vi "labpavi4.vi"() -> ()   [LabVIEW 2025]
uses:
  <vilib>/Analysis/3filter.llb/Filter Passband Type.ctl
  <vilib>/Analysis/2dsp.llb/Real FFT.vi
  <vilib>/Analysis/3filter.llb/Butterworth Filter (DBL).vi
  <vilib>/measure/NI_MABase.lvlib
  <vilib>/Analysis/NI_AALPro.lvlib
  <vilib>/Analysis/NI_AALBase.lvlib
panel:
  out "Waveform Graph 3":dbl[](graph)
  out "Waveform Graph":dbl[](graph)
  in  "samples":dbl=10.0 format="%0.2p"
  in  "sampfreq":dbl=10.0 format="%0.2p"
  out "Frequency label":waveform(dbl)(graph)
  out "spectrum":cluster{"Y":dbl[], "Y":dbl[]}[](graph)
  in  "deltaf":dbl
  out "Output":dbl[](graph)
  in  "fc":dbl
  out "Message":waveform(dbl)(graph)
  in  "fm":dbl=10.0 format="%0.2p"
  in  "am":dbl=1.0 format="%0.2p"
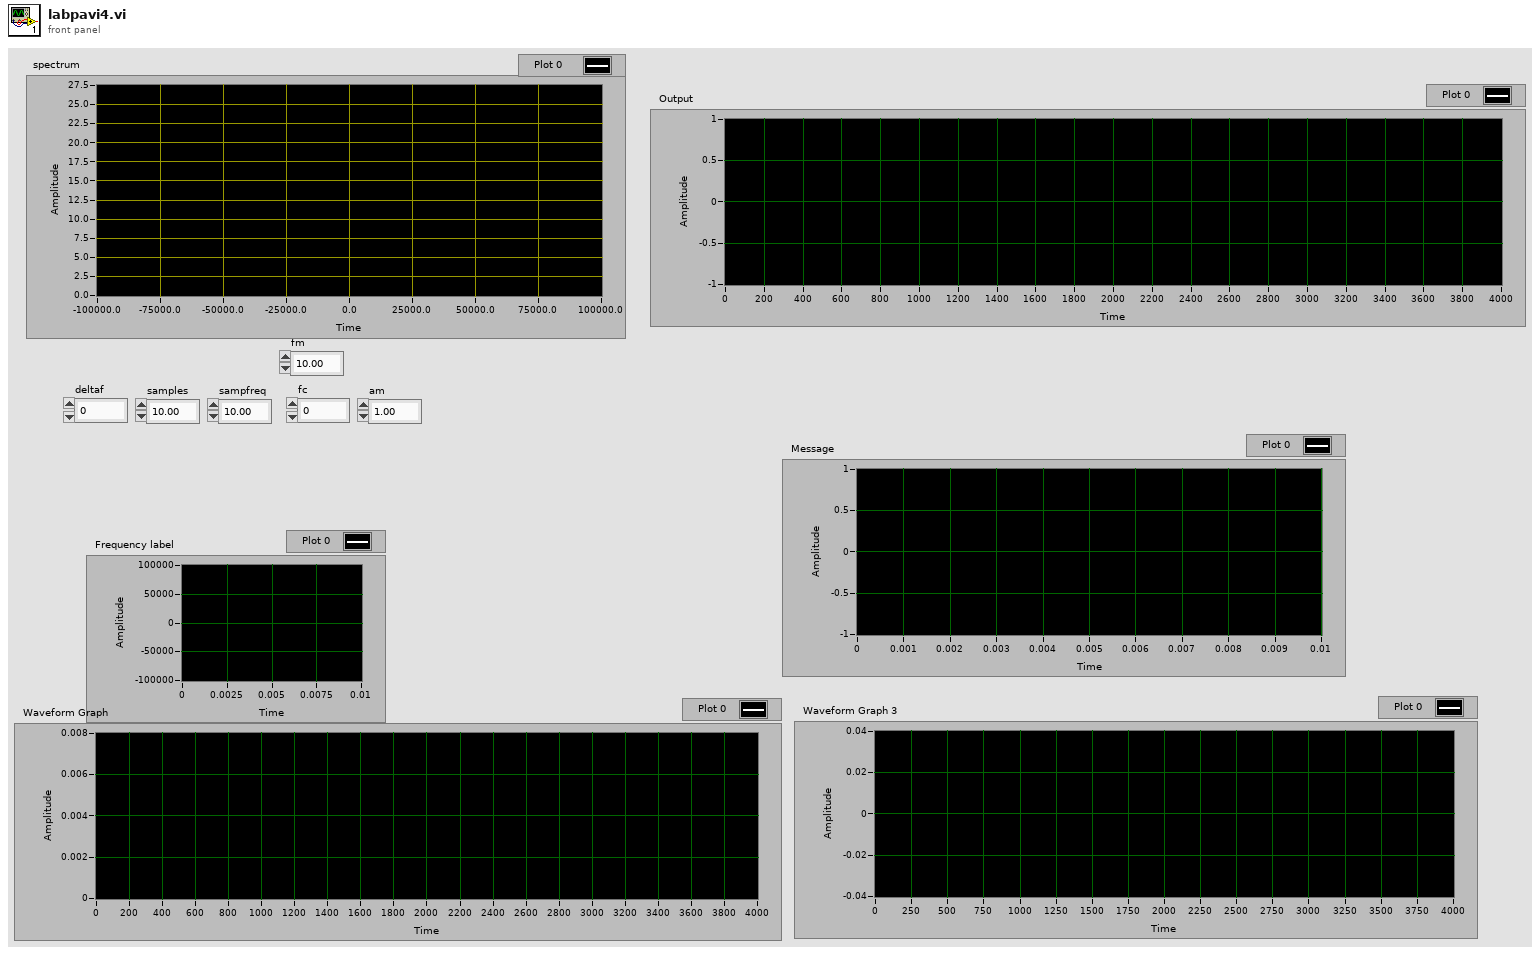
[diagram p1: front panel]
types:
  T1 = typedef "NI_AALBase.lvlib/Filter Passband Type.ctl" = enum32{"Lowpass", "Highpass", "Bandpass", "Bandstop"}
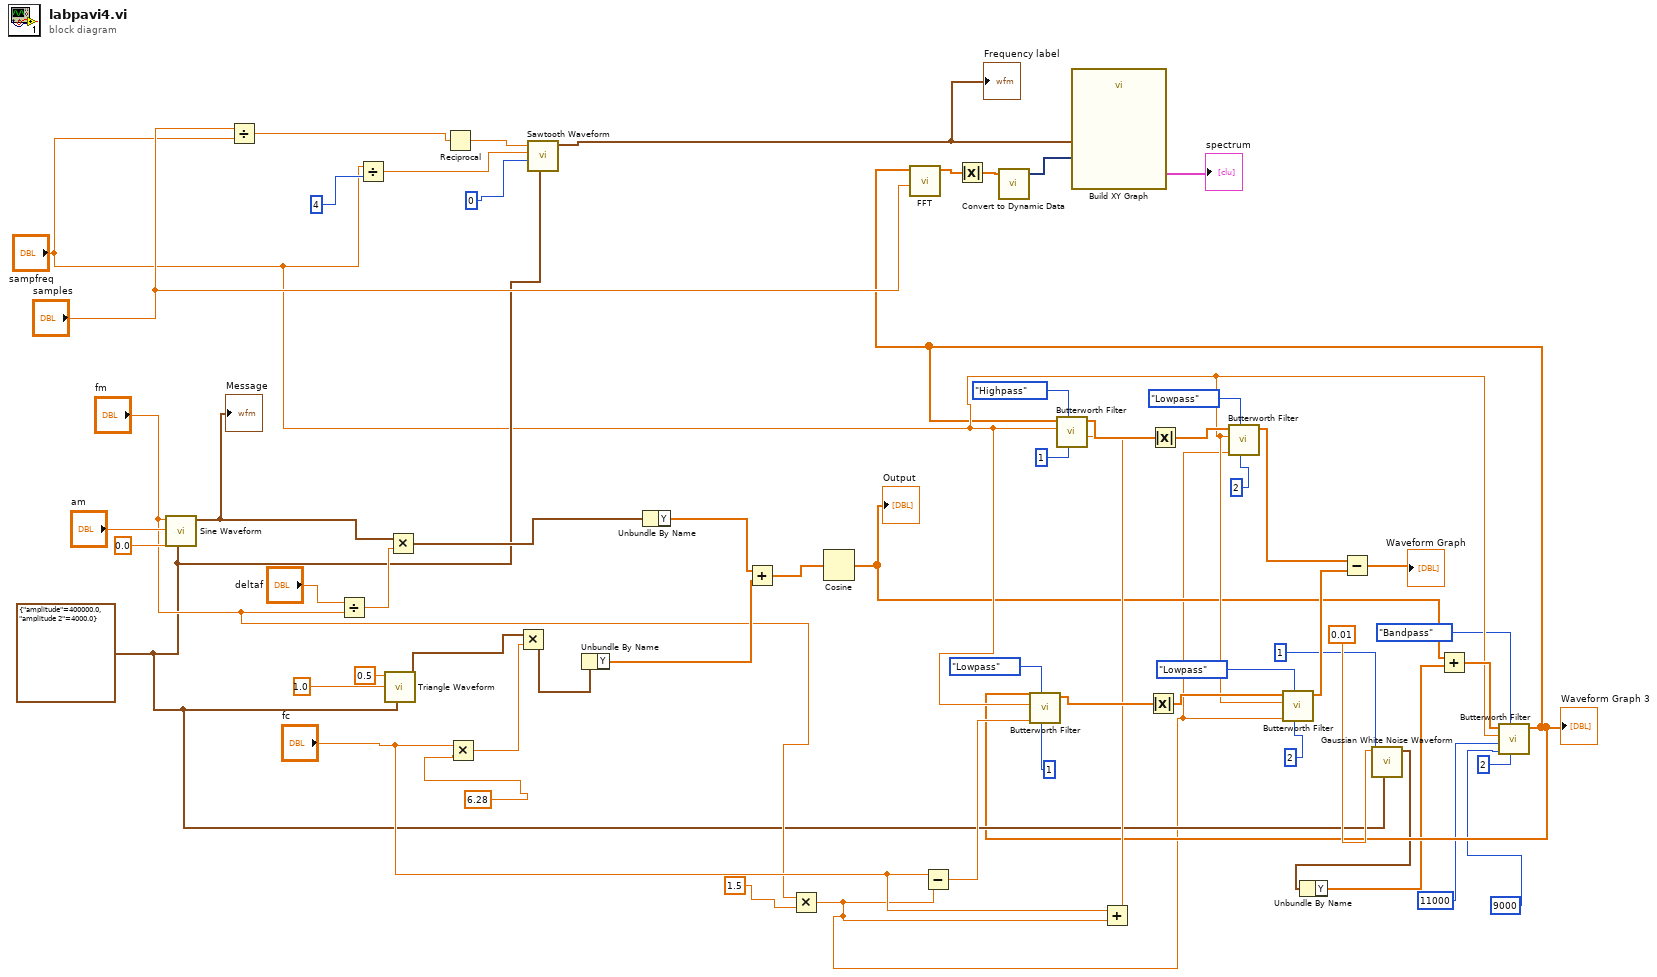
[diagram p0: block diagram]
diagram:
  w17 = cluster{"amplitude":dbl, "amplitude 2":dbl} {"amplitude"=400000.0, "amplitude 2"=4000.0}
  n1 = call <vilib>:"Sine Waveform.vi"("sampling info"=w17, "phase"=0.0, "amplitude"="am", "frequency"="fm") -> ("signal out"=w58:waveform(dbl))  [unwired: 6 in, 1 out]
  "Message" <- w58
  n2 = Divide(x="samples", y="sampfreq") -> (x/y=w46:dbl)
  n3 = Divide(x="deltaf", y="fm") -> (x/y=w57:dbl)
  n4 = Divide(x="sampfreq", y=4) -> (x/y=w47:dbl)
  n5 = call <vilib>:"Triangle Waveform.vi"("sampling info"=w17, "amplitude"=1.0, "frequency"=0.5) -> ("signal out"=w53:waveform(dbl))  [unwired: 7 in, 1 out]
  n6 = Multiply(x=w58, y=w57) -> (x*y=w50:waveform(dbl))
  n7 = Reciprocal(x=w46) -> (1/x=w45:dbl)
  n8 = Multiply(x="fc", y=6.28) -> (x*y=w54:dbl)
  n9 = Multiply(x=w53, y=w54) -> (x*y=w52:waveform(dbl))
  n10 = call <vilib>:"Sawtooth Waveform.vi"("sampling info"=w17, "phase"=0, "amplitude"=w47, "frequency"=w45) -> ("signal out"=w40:waveform(dbl))  [unwired: 6 in, 1 out]
  "Frequency label" <- w40
  n11 = Unbundle By Name(w52) -> ("Y"=w51:dbl[])
  n12 = Unbundle By Name(w50) -> ("Y"=w49:dbl[])
  n13 = Add(x=w49, y=w51) -> (x+y=w37:dbl[])
  n14 = Multiply(x="fm", y=1.5) -> (x*y=w4:dbl)
  n15 = Cosine(x=w37) -> (cos(x)=w9:dbl[])
  "Output" <- w9
  n16 = Subtract(x="fc", y=w4) -> (x-y=w28:dbl)
  n17 = Add(x="fc", y=w4) -> (x+y=w27:dbl)
  n18 = call <vilib>:"Gaussian White Noise Waveform.vi"("sampling info"=w17, "seed"=1, "standard deviation"=0.01) -> ("signal out"=w2:waveform(dbl))  [unwired: 7 in, 1 out]
  n19 = Unbundle By Name(w2) -> ("Y"=w1:dbl[])
  n20 = Add(x=w9, y=w1) -> (x+y=w12:dbl[])
  n21 = call-poly <vilib>:"Butterworth Filter.vi"("order"=2, "filter type"=Filter_Passband_Type."Bandpass", "low cutoff freq: fl"=9000, "high cutoff freq: fh"=11000, "sampling freq: fs"="sampfreq", "X"=w12) -> ("Filtered X"=w7:dbl[])  [unwired: 2 in, 1 out]
  "Waveform Graph 3" <- w7
  n22 = call-poly <vilib>:"FFT.vi"("FFT size"="samples", "X"=w7) -> ("FFT {X}"=w43:cdb[])  [unwired: 8 in, 1 out]
  n23 = Absolute Value(x=w43) -> (abs(x)=w39:dbl[])
  n24 = call "Convert to Dynamic Data"("Array"=w39) -> ("Dynamic Data Type"=w38:dynamicdata)  [unwired: 3 in]
  n25 = call-poly <vilib>:"Butterworth Filter.vi"("order"=1, "filter type"=Filter_Passband_Type."Lowpass", "low cutoff freq: fl"=w28, "sampling freq: fs"="sampfreq", "X"=w7) -> ("Filtered X"=w31:dbl[])  [unwired: 3 in, 1 out]
  n26 = call-poly <vilib>:"Butterworth Filter.vi"("order"=1, "filter type"=Filter_Passband_Type."Highpass", "high cutoff freq: fh"=w27, "sampling freq: fs"="sampfreq", "X"=w7) -> ("Filtered X"=w32:dbl[])  [unwired: 3 in, 1 out]
  n27 = call "Build XY Graph"("Y Input"=w38, "X Input"=w40) -> ("XY Graph"=→"spectrum":cluster{"X":dbl[], "Y":dbl[]}[])  [unwired: 8 in, 1 out]
  n28 = Absolute Value(x=w31) -> (abs(x)=w29:dbl[])
  n29 = Absolute Value(x=w32) -> (abs(x)=w30:dbl[])
  n30 = call-poly <vilib>:"Butterworth Filter.vi"("order"=2, "filter type"=Filter_Passband_Type."Lowpass", "low cutoff freq: fl"=w4, "sampling freq: fs"="sampfreq", "X"=w30) -> ("Filtered X"=w23:dbl[])  [unwired: 3 in, 1 out]
  n31 = call-poly <vilib>:"Butterworth Filter.vi"("order"=2, "filter type"=Filter_Passband_Type."Lowpass", "low cutoff freq: fl"=w4, "sampling freq: fs"="sampfreq", "X"=w29) -> ("Filtered X"=w22:dbl[])  [unwired: 3 in, 1 out]
  n32 = Subtract(x=w23, y=w22) -> (x-y=→"Waveform Graph":dbl[])
